vi "read_ini.vi"(8 "error in (no error)":errorcluster caption="错误输入（无错误）", 9 "section name":string, 10 "file ref in":T1, 11 "OneMotion 输入":refnum<class "OneMotion.lvclass">) -> (0 "error out":errorcluster caption="错误输出", 2 "file ref out":T1, 3 "OneMotion 输出":refnum<class "OneMotion.lvclass">)   [LabVIEW 2016, in "MotionControl_UFO_3DOF.lvlib" / "OneMotion.lvclass"]
uses:
  <userlib>/MotionControl_UFO_3DOF/OneMotion/OneMotion.lvclass
  <vilib>/Utility/config.llb/Config Data RefNum.ctl
  <userlib>/MotionControl_UFO_3DOF/OneMotion/hard limit option.ctl
  <userlib>/MotionControl_UFO_3DOF/OneMotion/unit mode.ctl
  <userlib>/MotionControl_UFO_3DOF/OneMotion/backlash option.ctl
  <userlib>/MotionControl_UFO_3DOF/OneMotion/OneMotion.lvclass/OneMotion.ctl
  <userlib>/MotionControl_UFO_3DOF/LimitSwitch/LimitSwitch.lvclass
  <vilib>/Utility/config.llb/Read Key (String).vi
  <vilib>/Utility/config.llb/Read Key (I32).vi
  <vilib>/Utility/config.llb/Read Key (Double).vi
  <vilib>/Utility/config.llb/Read Key (U32).vi
  <vilib>/ErrorRing/Error Ring.xnode
  <userlib>/MotionControl_UFO_3DOF/StepMotor/StepMotor.lvclass
  <vilib>/Utility/config.llb/NI_LVConfig.lvlib
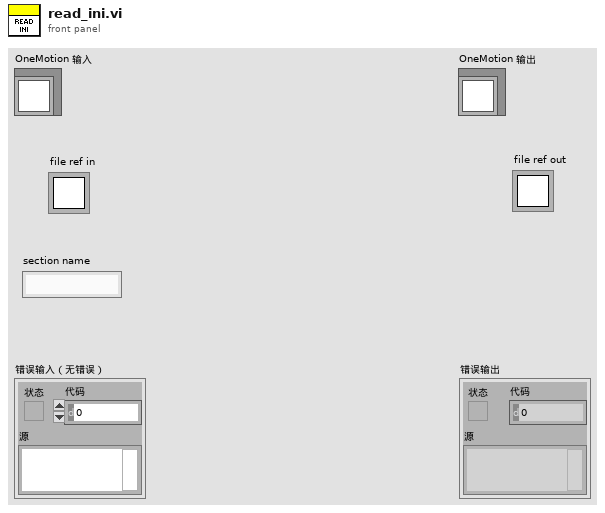
[diagram p1: front panel]
types:
  T1 = typedef "NI_LVConfig.lvlib/Config Data RefNum.ctl" = refnum<k1>
  T2 = typedef "MotionControl_UFO_3DOF.lvlib/OneMotion.lvclass/backlash option.ctl" = enum16{"no backlash compensation", "compensation: from - to +", "compensation: from + to -"}
  T3 = typedef "MotionControl_UFO_3DOF.lvlib/OneMotion.lvclass/unit mode.ctl" = enum16{"motor (pulse)", "linear (mm) or radial (degree)"}
  T4 = typedef "MotionControl_UFO_3DOF.lvlib/OneMotion.lvclass/hard limit option.ctl" = enum16{"STOP, and a 0.5s timeout constraint in move", "STOP, and move disabled"}
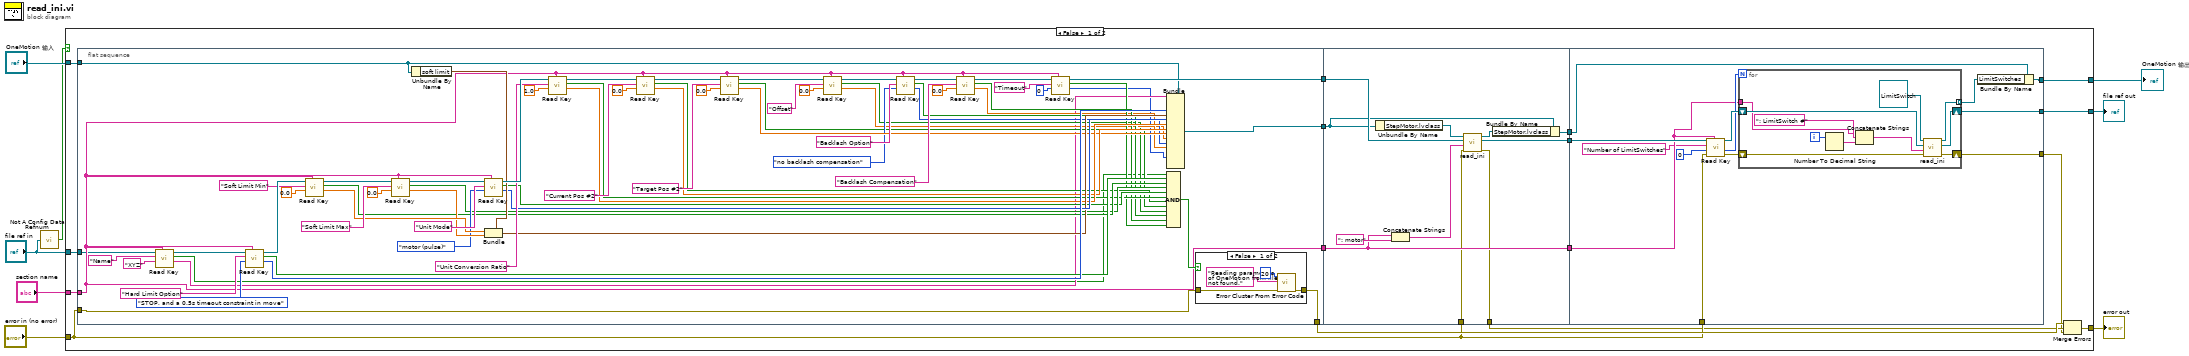
[diagram p0: block diagram]
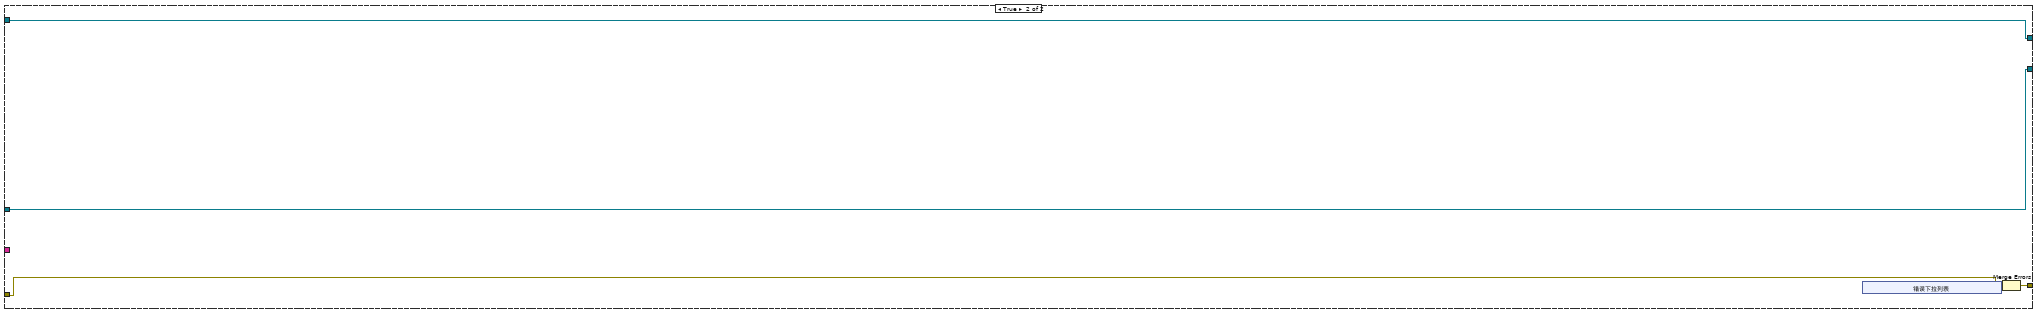
[diagram p3: hidden frame]
diagram:
  n1 = call <vilib>:"Not A Config Data Refnum.vi"("refnum"="file ref in") -> ("not a config data refnum"=w5:bool)
  n2 = case shown="False" w5 {
    tunnel: [w9 w135] -> w8
    tunnel: [w17 w138] -> w6
    tunnel: "OneMotion 输入" -> [w19 w138]
    tunnel: "error in (no error)" -> [w12 w136]
    tunnel: "file ref in" -> [w23 w134]
    tunnel: [w22 w134] -> w2
    tunnel: "section name" -> [w24 _]
    frame False {
      n3 = flat-sequence {
        tunnel: w23 -> [w29]
        tunnel: w24 -> [w31]
        tunnel: [w75] -> w21
        tunnel: [w31] -> w20
        tunnel: w19 -> [w72]
        tunnel: [w54] -> w18
        tunnel: w12 -> [w42]
        tunnel: [w41] -> w13
        tunnel: w21 -> [w108]
        tunnel: w20 -> [w101]
        tunnel: w18 -> [w104]
        tunnel: [w109] -> w16
        tunnel: [w102] -> w15
        tunnel: [w101] -> w14
        tunnel: w12 -> [w100]
        tunnel: [w99] -> w11
        tunnel: [w121] -> w17
        tunnel: [w119] -> w22
        tunnel: w16 -> [w118]
        tunnel: w15 -> [w122]
        tunnel: w14 -> [w111]
        tunnel: w12 -> [w113]
        tunnel: [w120] -> w10
        frame #0 {
          n4 = call-poly <vilib>:"Read Key.vi"("section"=w31, "default value"="XYZ", "key"="Name", "refnum"=w29) -> ("value"=w27:string, "found?"=w26:bool, "refnum out"=w30:T1)  [unwired: 4 in, 1 out]
          n5 = call-poly <vilib>:"Read Key.vi"("section"=w31, "default value"=hard_limit_option."STOP, and a 0.5s timeout constraint in move" ("hard limit option"), "key"="Hard Limit Option", "refnum"=w30) -> ("value"=w71:i32, "found?"=w53:bool, "refnum out"=w92:T1)  [unwired: 4 in, 1 out]
          n6 = call-poly <vilib>:"Read Key.vi"("section"=w31, "default value"=0.0, "key"="Soft Limit Min", "refnum"=w92) -> ("value"=w69:dbl, "found?"=w52:bool, "refnum out"=w91:T1)  [unwired: 4 in, 1 out]
          n7 = call-poly <vilib>:"Read Key.vi"("section"=w31, "default value"=0.0, "key"="Soft Limit Max", "refnum"=w91) -> ("value"=w68:dbl, "found?"=w51:bool, "refnum out"=w88:T1)  [unwired: 4 in, 1 out]
          n8 = Unbundle By Name(w72) -> ("soft limit"=w74:cluster{"min":dbl, "max":dbl})
          n9 = call-poly <vilib>:"Read Key.vi"("section"=w31, "default value"=unit_mode."motor (pulse)" ("unit mode"), "key"="Unit Mode", "refnum"=w88) -> ("value"=w65:i32, "found?"=w50:bool, "refnum out"=w87:T1)  [unwired: 4 in, 1 out]
          n10 = Bundle(cluster=w74, "min"=w69, "max"=w68) -> (w64:cluster{"min":dbl, "max":dbl})
          n11 = call-poly <vilib>:"Read Key.vi"("section"=w31, "default value"=1.0, "key"="Unit Conversion Ratio", "refnum"=w87) -> ("value"=w62:dbl, "found?"=w49:bool, "refnum out"=w86:T1)  [unwired: 4 in, 1 out]
          n12 = call-poly <vilib>:"Read Key.vi"("section"=w31, "default value"=0.0, "key"="Current Pos #2", "refnum"=w86) -> ("value"=w60:dbl, "found?"=w48:bool, "refnum out"=w82:T1)  [unwired: 4 in, 1 out]
          n13 = call-poly <vilib>:"Read Key.vi"("section"=w31, "default value"=0.0, "key"="Target Pos #2", "refnum"=w82) -> ("value"=w59:dbl, "found?"=w47:bool, "refnum out"=w37:T1)  [unwired: 4 in, 1 out]
          n14 = call-poly <vilib>:"Read Key.vi"("section"=w31, "default value"=0.0, "key"="Offset", "refnum"=w37) -> ("value"=w34:dbl, "found?"=w33:bool, "refnum out"=w36:T1)  [unwired: 4 in, 1 out]
          n15 = call-poly <vilib>:"Read Key.vi"("section"=w31, "default value"=backlash_option."no backlash compensation" ("backlash option"), "key"="Backlash Option", "refnum"=w36) -> ("value"=w39:i32, "found?"=w46:bool, "refnum out"=w81:T1)  [unwired: 4 in, 1 out]
          n16 = call-poly <vilib>:"Read Key.vi"("section"=w31, "default value"=0.0, "key"="Backlash Compensation", "refnum"=w81) -> ("value"=w40:dbl, "found?"=w45:bool, "refnum out"=w77:T1)  [unwired: 4 in, 1 out]
          n17 = call-poly <vilib>:"Read Key.vi"("section"=w31, "default value"=u32 0, "key"="Timeout", "refnum"=w77) -> ("value"=w25:u32, "found?"=w44:bool, "refnum out"=w75:T1)  [unwired: 4 in, 1 out]
          n18 = Bundle(cluster=w72, w27, w71, w64, w65, w62, w60, w59, w34, w39, w40, w25) -> (w54:refnum<class "OneMotion.lvclass">)  [unwired: 5 in]
          n19 = Compound Arithmetic op=AND(w26, w53, w52, w51, w50, w49, w48, w47, w33, w46, w45, w44) -> (w43:bool)
          n20 = case shown="False" w43 {
            tunnel: w42 -> [w95 w98]
            tunnel: [w94 w98] -> w41
            frame False {
              n21 = call <vilib>:"Error Cluster From Error Code.vi"("error in (no error)"=w95, "error message (\"\")"="Reading parameters of OneMotion from file not found." ("error message (\"\")"), "error code (0)"=20) -> ("error out"=w94:errorcluster)  [unwired: 6 in]
            }
            frame True {
            }
          }
        }
        frame #1 {
          n22 = Unbundle By Name(w104) -> ("StepMotor.lvclass"=w105:refnum<class "StepMotor.lvclass">)
          n23 = Concatenate Strings(w101, ": motor") -> (w106:string)
          n24 = call-dynamic "read_ini.vi"("error in (no error)"=w100, "section name"=w106, "file ref in"=w108, "StepMotor 输入"=w105) -> ("error out"=w99:errorcluster, "file ref out"=w109:T1, "StepMotor 输出"=w103:refnum<class "StepMotor.lvclass">)  [unwired: 5 in]
          n25 = Bundle By Name(cluster=w104, "StepMotor.lvclass"=w103) -> (w102:refnum<class "OneMotion.lvclass">)
        }
        frame #2 {
          n26 = call-poly <vilib>:"Read Key.vi"("section"=w111, "error in (no error)"=w113, "default value"=u32 0, "key"="Number of LimitSwitches", "refnum"=w118) -> ("error out"=w112:errorcluster, "value"=w115:u32, "refnum out"=w117:T1)  [unwired: 3 in, 1 out]
          n27 = for {
            N: w115 -> [_]
            shift-right: [w132] -> w119
            shift-left: w117 -> [w133]
            tunnel: w111 -> [w130]
            tunnel: [w127] -> w114 mode=indexing
            shift-right: [w125] -> w120
            shift-left: w112 -> [w126]
            i -> [w124]
            n28 = Number To Decimal String(number=w124) -> (decimal integer string=w129:string)  [unwired: 1 in]
            n29 = Concatenate Strings(w130, ": LimitSwitch #", w129) -> (w128:string)
            n30 = call-dynamic "read_ini.vi"("error in (no error)"=w126, "section name"=w128, "file ref in"=w133, "LimitSwitch 输入"=refnum<class "LimitSwitch.lvclass"> refnum) -> ("error out"=w125:errorcluster, "file ref out"=w132:T1, "LimitSwitch 输出"=w127:refnum<class "LimitSwitch.lvclass">)  [unwired: 5 in]
          }
          n31 = Bundle By Name(cluster=w122, "LimitSwitches"=w114) -> (w121:refnum<class "OneMotion.lvclass">)
        }
      }
      n32 = Merge Errors(w13, w11, w10) -> (w9:errorcluster)
    }
    frame True {
      n33 = xnode "错误下拉列表"() -> ("error out"=w137:errorcluster)
      n34 = Merge Errors(w136, w137) -> (w135:errorcluster)
    }
  }
  "error out" <- w8
  "OneMotion 输出" <- w6
  "file ref out" <- w2
